vi "Enable_channel_Integration_board_L1.vi"(1 "Combination":u8 max=127 step=1 format="%b", 2 "Enable  L1 single  Input":i32(slide) scale=0.0..6.0, 4 "error in (no error)":errorcluster, 5 "SingleIN/#Combination":bool, 6 "Enable some/all":bool, 7 "connection ID":refnum<k5>) -> (0 "error out":errorcluster, 3 "connection ID out":refnum<k5>)   [LabVIEW 2012]
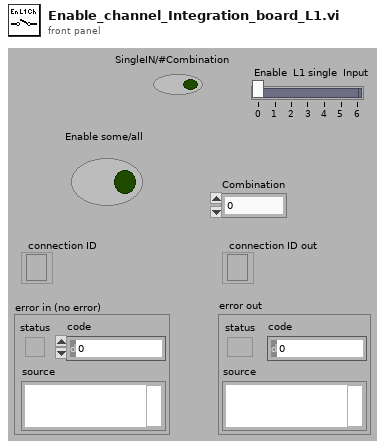
[diagram p1: front panel]
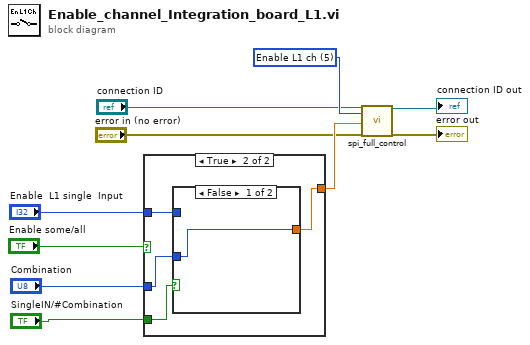
[diagram p0: block diagram]
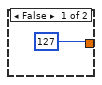
[diagram p2: hidden frame]
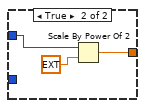
[diagram p3: hidden frame]
diagram:
  w8 = u16 5 items=["Attenuation", "Clipping", "Enable channel", "Delay line", "ASIC", "Enable L1 ch", "ASIC L1"] ("Device")
  n1 = case shown="True" "Enable some/all" {
    tunnel: [127 ("Register or channel") w14] -> w9
    tunnel: "Enable  L1 single  Input" -> [_ w15]
    tunnel: "Combination" -> [_ w13]
    tunnel: "SingleIN/#Combination" -> [_ w12]
    frame False {
    }
    frame True {
      n2 = case shown="False" w12 {
        tunnel: w15 -> [_ w18]
        tunnel: [w16 w17] -> w14
        tunnel: w13 -> [w16 _]
        frame False {
        }
        frame True {
          n3 = Scale By Power Of 2(n=w18, x=ext 1.0) -> (x*2^n=w17:ext)
        }
      }
    }
  }
  n4 = call "spi_full_control.vi"("connection ID"="connection ID", "Device"=w8, "Data"=w9, "error out 3"="error in (no error)") -> ("connection ID out"=→"connection ID out":refnum<k5>, "error out 2"=→"error out":errorcluster)  [unwired: 8 in, 6 out]
